vi "Control Path.vi"(11 "DblNumericStatusEditorPanel in":refnum<class "DblNumericStatusEditorPanel.lvclass">) -> (2 "Control Paths":path[](array[path]))   [LabVIEW 2020, in "VolatusGUIControls.lvlib" / "DblNumericStatusEditorPanel.lvclass"]
uses:
  DblNumericStatusEditorPanel.lvclass
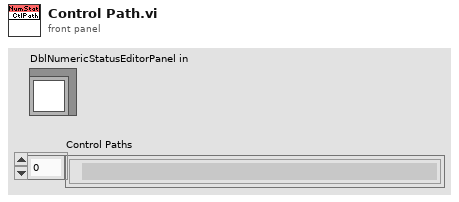
[diagram p1: front panel]
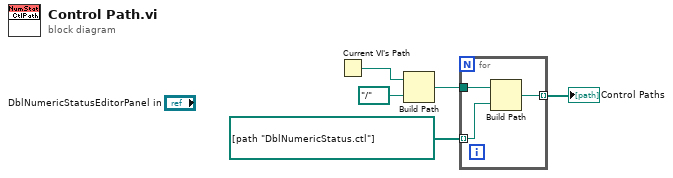
[diagram p0: block diagram]
diagram:
  n1 = Current VI's Path() -> (path=w5:path)
  n2 = Build Path(base path=w5, name or relative path=path "../..") -> (appended path=w3:path)
  n3 = for {
    tunnel: w3 -> [w8]
    tunnel: path[] [path "DblNumericStatus.ctl"] -> [w7] mode=indexing
    tunnel: [w6] -> w1 mode=indexing
    n4 = Build Path(base path=w8, name or relative path=w7) -> (appended path=w6:path)
  }
  "Control Paths" <- w1
